vi "LedBlink.vi"() -> ()   [LabVIEW 2020]
uses:
  <vilib>/MakerHub/LINX/Public/Peripherals/Digital/Digital Write 1 Chan.vi
  <vilib>/MakerHub/LINX/Public/Peripherals/Digital/Digital Write N Chans.vi
  <vilib>/MakerHub/LINX/Private/Local IO/LinxDigitalWrite.vi
  <vilib>/MakerHub/LINX/Public/Utilities/Check Channel.vi
  <vilib>/MakerHub/LINX/Public/Utilities/Open Serial.vi
  <vilib>/MakerHub/LINX/Private/Utilties/Generate Error.vi
  <vilib>/MakerHub/LINX/LMH-LINX.lvlib
panel:
  out "Device Name":string
  in  "stop":bool
  out "Boolean":bool
  in  "Slide":dbl(slide) scale=0.0..10.0
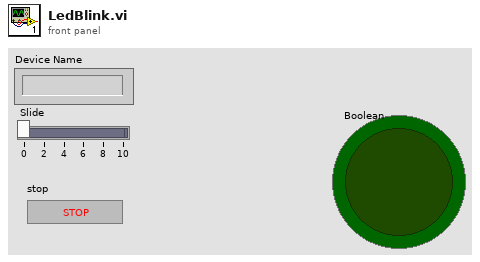
[diagram p1: front panel]
types:
  T1 = typedef "LMH-LINX.lvlib/LINX Ref.ctl" = cluster{"IO":T2, "Interface":T3, "LINX Device Config":T4}
  T2 = typedef "LMH-LINX.lvlib/Platform.ctl" = enum16{"Remote", "Local"}
  T3 = typedef "LMH-LINX.lvlib/Interface.ctl" = enum16{"Serial", "TCP"}
  T4 = typedef "LMH-LINX.lvlib/Device.lvlib/LINX Device Config.ctl" = cluster{"Interface":T3, "COM Port":refnum<visa-resource-name>, "TCP Configuration":T5, "Device Family":u8, "Device ID":u8, "Device Name":string, "TCP Ref":refnum<k5>, "Channels":T6}
  T5 = typedef "LMH-LINX.lvlib/Device.lvlib/TCP Config.ctl" = cluster{"IP Address":string, "Port":u16}
  T6 = typedef "LMH-LINX.lvlib/Channels.ctl" = cluster{"DI":u8[], "DO":u8[], "AI":u8[], "AO":u8[], "PWM":u8[], "QE":u8[], "UART":u8[], "I2C 2":u8[], "SPI":u8[], "CAN":u8[], "Servo":u8[], "AI Ref (V)":dbl, "AI Resolution (Bits)":u8, "AO Ref (V)":dbl, "AO Resolution (Bits)":u8}
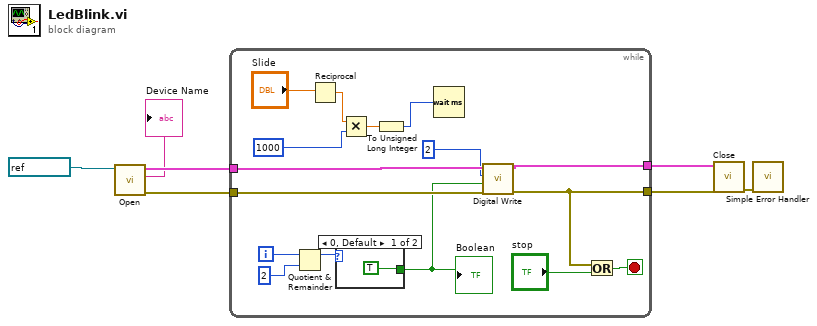
[diagram p0: block diagram]
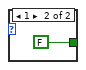
[diagram p2: hidden frame]
diagram:
  n1 = call-poly <vilib>:"Open.vi"("Serial Port"=refnum<visa-resource-name> "COM3") -> ("Error Out"=w5:errorcluster, "Device Name"=→"Device Name":string, "LINX Resource"=w7:T1)  [unwired: 8 in]
  n2 = while {
    tunnel: w7 -> [w18]
    tunnel: [w17] -> w6
    tunnel: w5 -> [w15]
    tunnel: [w10] -> w4
    i -> [w13]
    stop <- w8 stop-if-true
    n3 = Quotient & Remainder(x=w13, y=2) -> (x-y*floor(x/y)=w14:i32)  [unwired: 1 out]
    n4 = Reciprocal(x="Slide") -> (1/x=w22:dbl)
    n5 = case shown="0, Default" w14 {
      tunnel: [TRUE FALSE] -> w11
      frame 0, Default {
      }
      frame 1 {
      }
    }
    "Boolean" <- w11
    n6 = Multiply(x=w22, y=u32 1000 ("millisecond timer value")) -> (x*y=w20:dbl)
    n7 = To Unsigned Long Integer(number=w20) -> (unsigned 32bit integer=w19:u32)
    n8 = Wait (ms)(milliseconds to wait=w19) -> ()  [unwired: 1 out]
    n9 = call-poly <vilib>:"Digital Write.vi"("Error In"=w15, "Output Value"=w11, "DO Channel"=u8 2, "LINX Resource"=w18) -> ("Error Out"=w10:errorcluster, "LINX Resource"=w17:T1)  [unwired: 6 in]
    n10 = Or(x=w10, y="stop") -> (x .or. y?=w8:bool)
  }
  n11 = call <vilib>:"Close.vi"("Error In"=w4, "LINX Resource"=w6) -> ("Error Out"=w3:errorcluster)  [unwired: 9 in]
  n12 = call <vilib>:"Simple Error Handler.vi"("error in (no error)"=w3) -> ()  [unwired: 4 in, 5 out]
